vi "JTAG String to String.vi"() -> ()   [LabVIEW 2010]
panel:
  in  "Boolean":bool=TRUE
  out "String Out":string
  out "Array 2":string[][](array[string])
  out "Array 1":string[][](array[string])
  in  "String":string
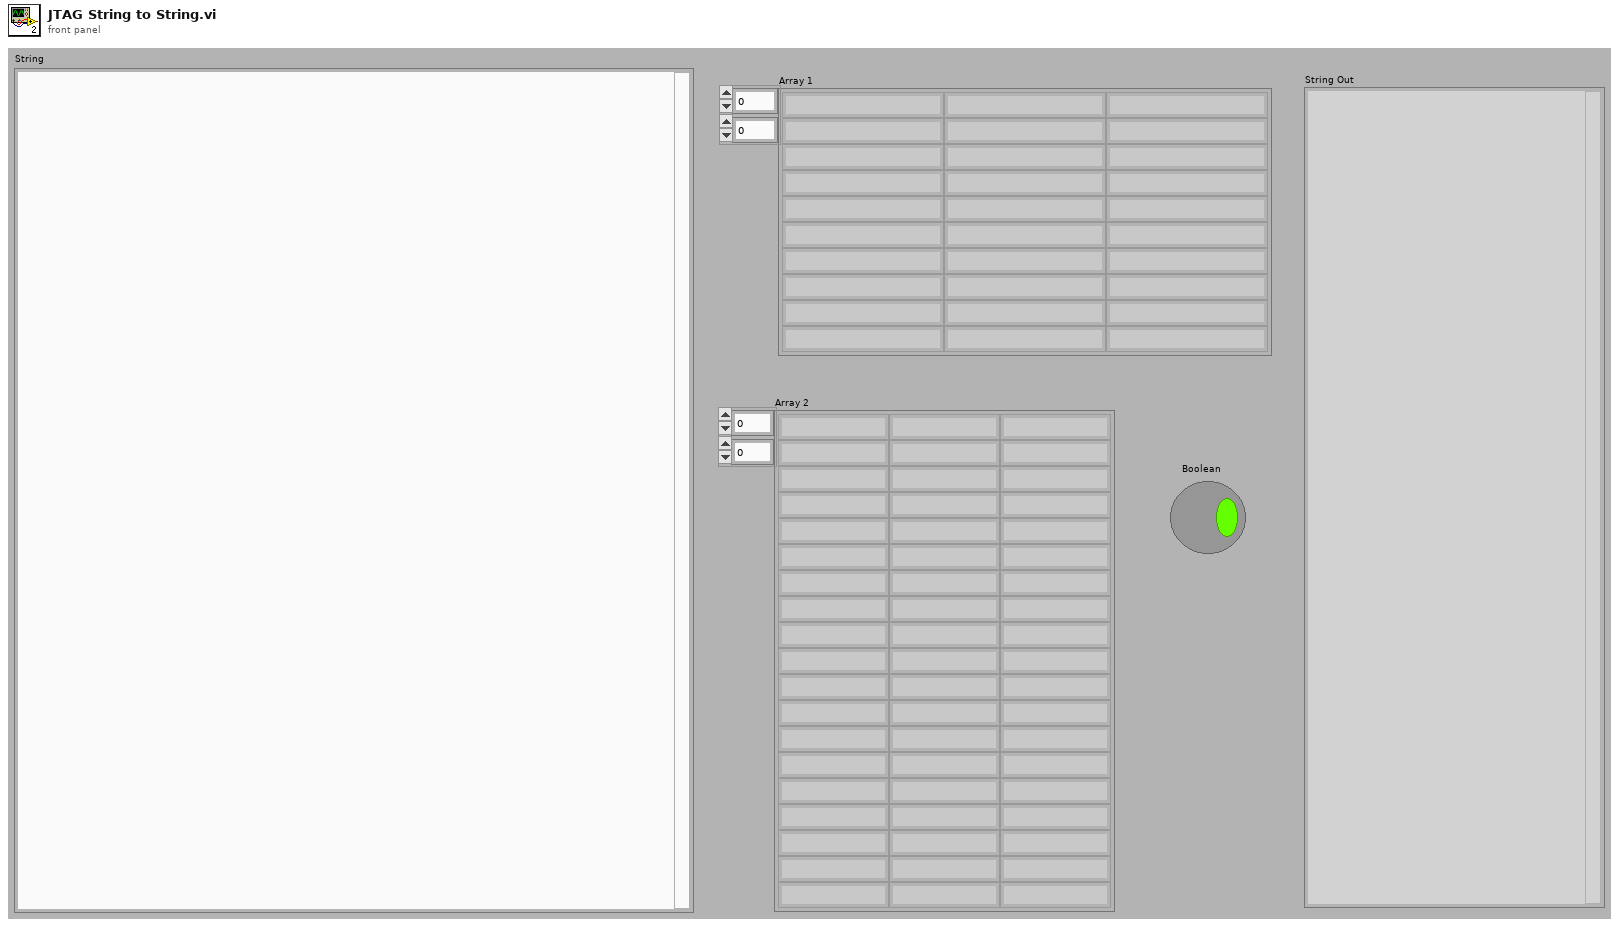
[diagram p1: front panel]
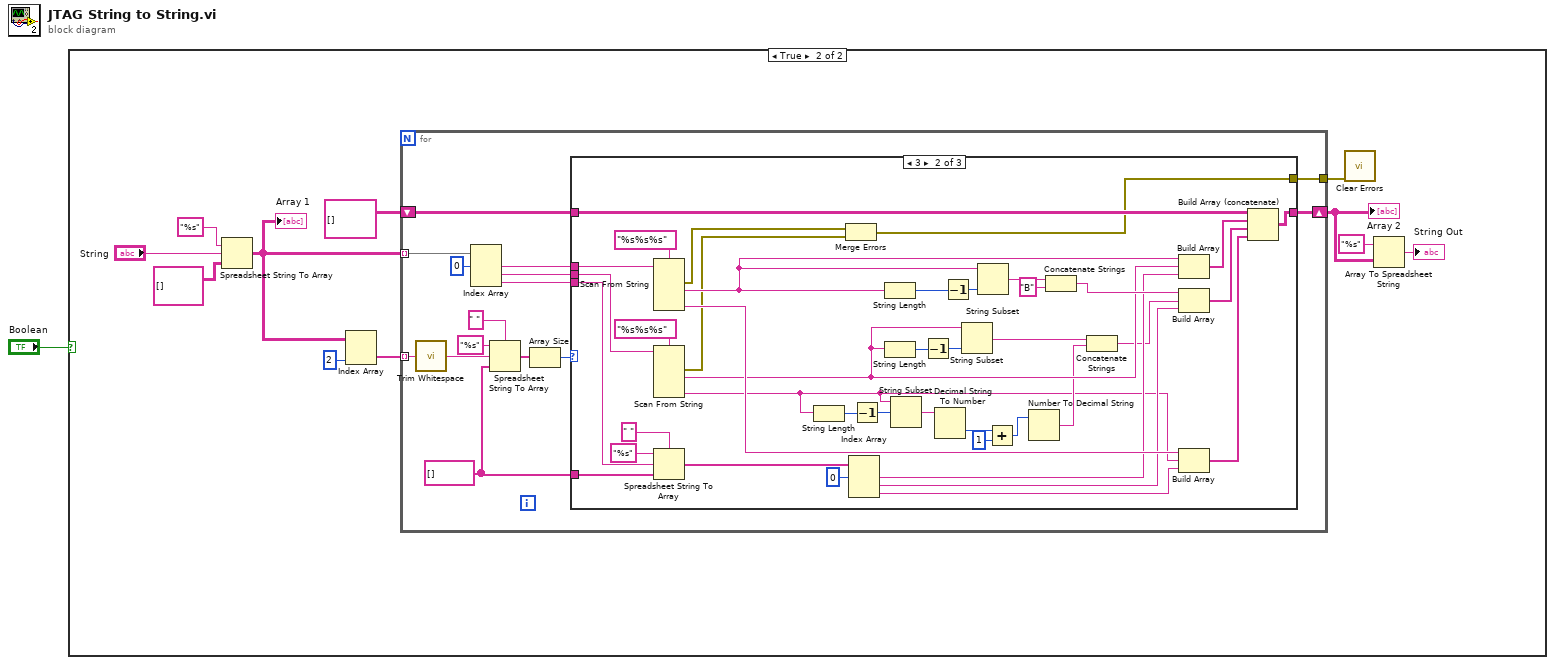
[diagram p0: block diagram]
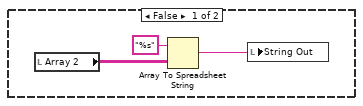
[diagram p2: hidden frame]
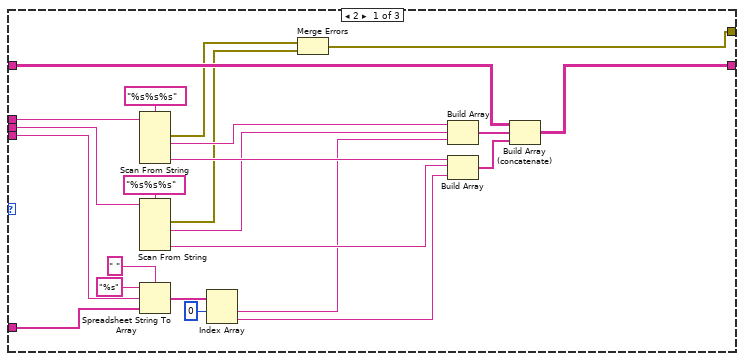
[diagram p3: hidden frame]
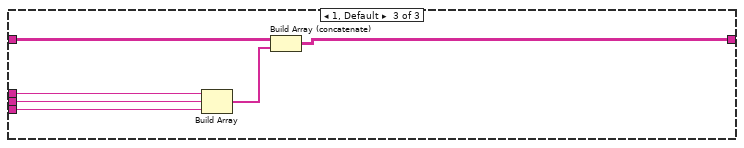
[diagram p4: hidden frame]
diagram:
  n1 = case shown="True" "Boolean" {
    frame False {
      n2 = local read "Array 2"() -> (w3:string[][])
      n3 = Array To Spreadsheet String(array=w3, 3:"%s" ("format string")) -> (spreadsheet string=w4:string)  [unwired: 1 in]
      n4 = local write "String Out"(w4) -> ()
    }
    frame True {
      n5 = Spreadsheet String To Array(format string="%s" ("spreadsheet string"), spreadsheet string="String", array type (2D Dbl)=string[][] []) -> (array=w6:string[][])  [unwired: 1 in]
      "Array 1" <- w6
      n6 = Index Array(array=w6, index (col)=2 ("disabled index (col)")) -> (element=w11:string[])  [unwired: 1 in]
      n7 = for {
        tunnel: w11 -> [w26] mode=indexing
        tunnel: w6 -> [w21] mode=indexing
        shift-right: [w25] -> w9
        shift-left: string[][] [] -> [w24]
        tunnel: [w16] -> w5
        w23 = string[] [] ("array type (2D Dbl)")
        n8 = call <vilib>:"Trim Whitespace.vi"("string"=w26) -> ("trimmed string"=w17:string)  [unwired: 1 in]
        n9 = Index Array(array=w21, index #1=0 ("index")) -> (element #1=w20:string, element #2=w19:string, element #3=w18:string)  [unwired: 2 in]
        n10 = Spreadsheet String To Array(delimiter (Tab)=" ", format string="%s", spreadsheet string=w17, array type (2D Dbl)=w23) -> (array=w28:string[])
        n11 = Array Size(array=w28) -> (size(s)=w27:i32)
        n12 = case shown="3" w27 {
          tunnel: [w48 w90 w100] -> w25
          tunnel: w24 -> [w44 w88 w99]
          tunnel: w23 -> [w43 w87 _]
          tunnel: w20 -> [w42 w59 w97]
          tunnel: w19 -> [w41 w58 w96]
          tunnel: w18 -> [w40 w57 w95]
          tunnel: [w31 w54 _] -> w16
          frame 2 {
            n13 = Scan From String(format string="%s%s%s", input string=w42) -> (error out=w33:errorcluster, output 1=w39:string, output 3=w38:string)  [unwired: 6 in, 2 out]
            n14 = Scan From String(format string="%s%s%s", input string=w41) -> (error out=w32:errorcluster, output 1=w37:string, output 3=w36:string)  [unwired: 6 in, 2 out]
            n15 = Spreadsheet String To Array(delimiter (Tab)=" ", format string="%s", spreadsheet string=w40, array type (2D Dbl)=w43) -> (array=w47:string[])
            n16 = Index Array(array=w47, index #1=0 ("index")) -> (element #1=w35:string, element #2=w34:string)  [unwired: 1 in]
            n17 = Merge Errors(w33, w32) -> (w31:errorcluster)
            n18 = Build Array(w39, w37, w35) -> (w51:string[])
            n19 = Build Array(w38, w36, w34) -> (w45:string[])
            n20 = Build Array (concatenate)(w44, w51, w45) -> (w48:string[][])
          }
          frame 3 {
            n21 = Scan From String(format string="%s%s%s", input string=w59) -> (error out=w56:errorcluster, output 1=w76:string, output 3=w78:string)  [unwired: 6 in, 2 out]
            n22 = Scan From String(format string="%s%s%s", input string=w58) -> (error out=w55:errorcluster, output 1=w71:string, output 3=w60:string)  [unwired: 6 in, 2 out]
            n23 = Spreadsheet String To Array(delimiter (Tab)=" ", format string="%s", spreadsheet string=w57, array type (2D Dbl)=w87) -> (array=w89:string[])
            n24 = String Length(string=w60) -> (length=w67:i32)
            n25 = Merge Errors(w56, w55) -> (w54:errorcluster)
            n26 = Index Array(array=w89, index #1=0 ("index")) -> (element #1=w73:string, element #2=w74:string, element #3=w75:string)  [unwired: 2 in]
            n27 = Decrement(x=w67) -> (x-1=w66:i32)
            n28 = String Length(string=w76) -> (length=w85:i32)
            n29 = String Length(string=w71) -> (length=w72:i32)
            n30 = String Subset(string=w60, offset (0)=w66) -> (substring=w65:string)  [unwired: 1 in]
            n31 = Decrement(x=w72) -> (x-1=w70:i32)
            n32 = Decimal String To Number(string=w65) -> (number=w64:i32)  [unwired: 2 in, 1 out]
            n33 = Decrement(x=w85) -> (x-1=w84:i32)
            n34 = String Subset(string=w71, length (rest)=w70) -> (substring=w69:string)  [unwired: 1 in]
            n35 = String Subset(string=w76, length (rest)=w84) -> (substring=w81:string)  [unwired: 1 in]
            n36 = Add(x=w64, y=1) -> (x+y=w62:i32)
            n37 = Number To Decimal String(number=w62) -> (decimal integer string=w61:string)  [unwired: 1 in]
            n38 = Concatenate Strings(w81, "B" ("string")) -> (w79:string)
            n39 = Concatenate Strings(w69, w61) -> (w68:string)
            n40 = Build Array(w76, w71, w73) -> (w83:string[])
            n41 = Build Array(w79, w68, w74) -> (w82:string[])
            n42 = Build Array(w78, w60, w75) -> (w77:string[])
            n43 = Build Array (concatenate)(w88, w83, w82, w77) -> (w90:string[][])
          }
          frame 1, Default {
            n44 = Build Array(w97, w96, w95) -> (w98:string[])
            n45 = Build Array (concatenate)(w99, w98) -> (w100:string[][])
          }
        }
      }
      "Array 2" <- w9
      n46 = call <vilib>:"Clear Errors.vi"("error in (no error)"=w5) -> ()  [unwired: 6 in, 1 out]
      n47 = Array To Spreadsheet String(array=w9, 3:"%s" ("format string")) -> (spreadsheet string=→"String Out":string)  [unwired: 1 in]
    }
  }
